vi "AIT 664 - ReadWrite All Data.vi"(0 "RT Data in":T2 {"End System Handle" format="%x"; "Label Transfer Config"."Block Data Refs"."Data Reference" format="%.0x"; "Status Config"."Hardware Out Dur Reference" format="%.0x"; "Status Config"."Hardware In Dur Reference" format="%.0x"; "Status Config"."Hardware Out Count Reference" format="%.0x"; "Status Config"."Hardware In Count Reference" format="%.0x"; "Status Config"."Error Data Reference" format="%.0x"; "Hardware Output Tx Channels"."Message Settings"."Transmit Channel Data Reference" format="%.0x"; "Hardware Output Tx Channels"."Message Settings"."Queue Transmit Channel" format="%.0x"; "Hardware Output Tx Channels"."Message Settings"."Driver Data"."Num Bits" min=1 max=32; "Hardware Output Tx Channels"."Message Settings"."Block Data Refs"."Data Reference" format="%.0x"; "Hardware Output Tx Channels"."Rx Com Udp Port"."Handle" format="%08x"; "Hardware Output Tx Channels"."Tx Com Udp Port"."Handle" format="%08x"; "Hardware Input Rx Channels"."Message Settings"."Transmit Channel Data Reference" format="%.0x"; "Hardware Input Rx Channels"."Message Settings"."Queue Transmit Channel" format="%.0x"; "Hardware Input Rx Channels"."Message Settings"."Driver Data"."Num Bits" min=1 max=32; "Hardware Input Rx Channels"."Message Settings"."Block Data Refs"."Data Reference" format="%.0x"; "Hardware Input Rx Channels"."Rx Com Udp Port"."Handle" format="%08x"; "Hardware Input Rx Channels"."Tx Com Udp Port"."Handle" format="%08x"}, 2 "Mode":T1, 5 "Channel Index":i32, 11 "error in (no error)":errorcluster, 12 "Iteration":i32) -> (4 "RT Data out":T2 {"End System Handle" format="%x"; "Label Transfer Config"."Block Data Refs"."Data Reference" format="%.0x"; "Status Config"."Hardware Out Dur Reference" format="%.0x"; "Status Config"."Hardware In Dur Reference" format="%.0x"; "Status Config"."Hardware Out Count Reference" format="%.0x"; "Status Config"."Hardware In Count Reference" format="%.0x"; "Status Config"."Error Data Reference" format="%.0x"; "Hardware Output Tx Channels"."Message Settings"."Transmit Channel Data Reference" format="%.0x"; "Hardware Output Tx Channels"."Message Settings"."Queue Transmit Channel" format="%.0x"; "Hardware Output Tx Channels"."Message Settings"."Driver Data"."Num Bits" min=1 max=32; "Hardware Output Tx Channels"."Message Settings"."Block Data Refs"."Data Reference" format="%.0x"; "Hardware Output Tx Channels"."Rx Com Udp Port"."Handle" format="%08x"; "Hardware Output Tx Channels"."Tx Com Udp Port"."Handle" format="%08x"; "Hardware Input Rx Channels"."Message Settings"."Transmit Channel Data Reference" format="%.0x"; "Hardware Input Rx Channels"."Message Settings"."Queue Transmit Channel" format="%.0x"; "Hardware Input Rx Channels"."Message Settings"."Driver Data"."Num Bits" min=1 max=32; "Hardware Input Rx Channels"."Message Settings"."Block Data Refs"."Data Reference" format="%.0x"; "Hardware Input Rx Channels"."Rx Com Udp Port"."Handle" format="%08x"; "Hardware Input Rx Channels"."Tx Com Udp Port"."Handle" format="%08x"}, 15 "error out":errorcluster)   [LabVIEW 2013, in "AIT 664 Custom Device.lvlib"]
doc: "Given the mode provide either the hardware input or output channels to read/write from hardware or read/write to veristand."
uses:
  AIT 664 Custom Device.lvlib
  RT Controls/AIT 664  - RT Data.ctl
  RT Controls/AIT 664 - RT Hardware Channel.ctl
  RT Controls/AIT 664 - RT Message Settings.ctl
  <vilib>/NI Veristand/Custom Device API/Block Data Reference.ctl
  <vilib>/NI Veristand/Custom Device API/Data Reference.ctl
  RT Controls/AIT 664 - Driver Data.ctl
  Controls and Global/Start Bit.ctl
  Controls and Global/Number of Bits.ctl
  <vilib>/NI Veristand/Custom Device API/Custom Device Item Ref.ctl
  <userlib>/ARINC 664/AIT 664 Controls/General/Message Port.ctl
  <userlib>/ARINC 664/AIT 664 Controls/General/Direction.ctl
  <userlib>/ARINC 664/AIT 664 Controls/General/Message Port Type.ctl
  System Explorer/Controls/664 - Sampling Type.ctl
  RT Controls/Status Channels Config.ctl
  RT Controls/FIFO.ctl
  RT Controls/Label Transfer Config.ctl
  RT Controls/ReadWrite Selector.ctl
  <vilib>/NI Veristand/Custom Device API/Custom Device API.lvlib
  <userlib>/ARINC 664/AIT 664 API.lvlib
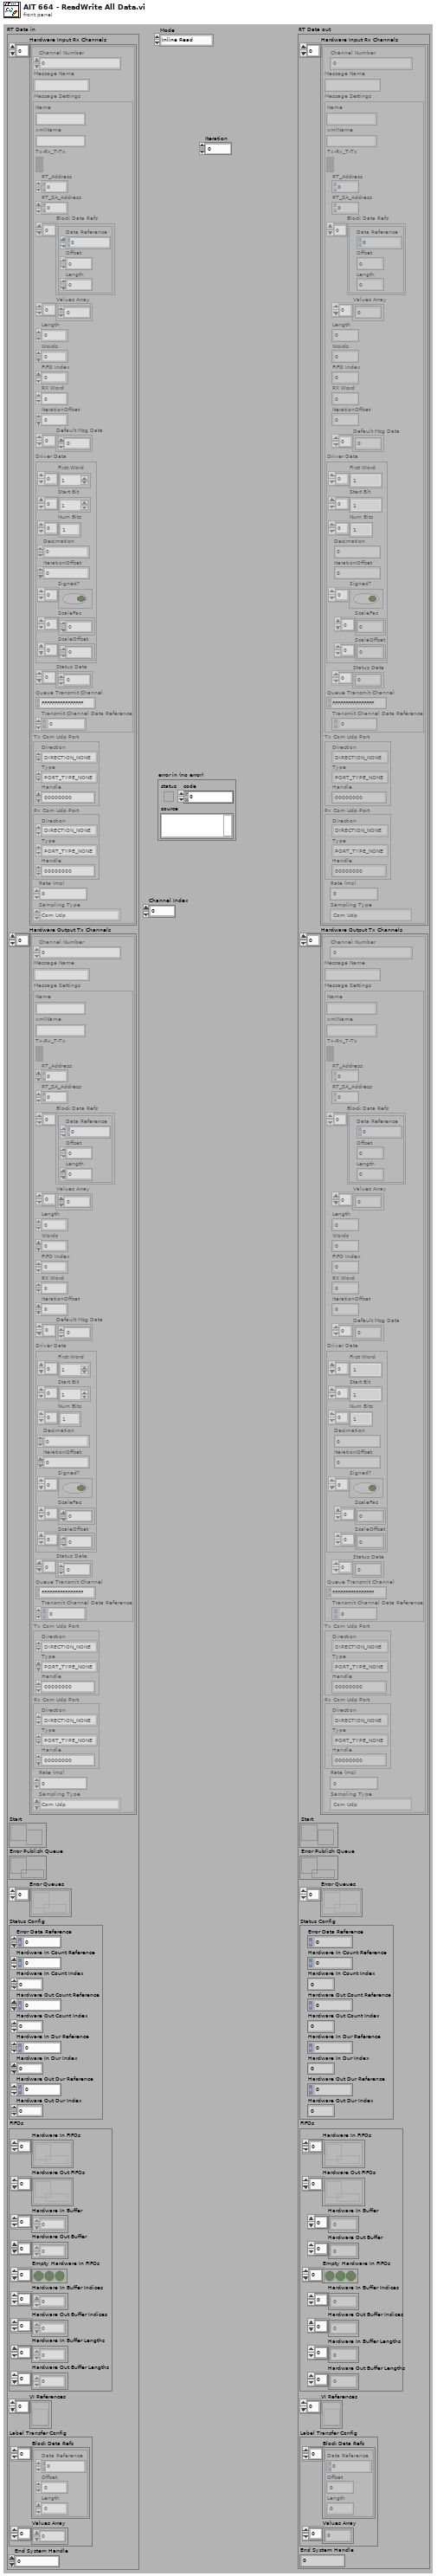
[diagram p1: front panel]
types:
  T1 = typedef "AIT 664 Custom Device.lvlib/ReadWrite Selector.ctl" = enum16{"Inline Read", "Inline Write", "Async HWIn", "Async HWOut"}
  T2 = typedef "AIT 664 Custom Device.lvlib/AIT 664  - RT Data.ctl" = cluster{"Hardware Input Rx Channels":T3[], "Hardware Output Tx Channels":T3[], "Start":refnum<notifier>, "Error Publish Queue":refnum<queue>, "Error Queues":refnum<queue>[], "Status Config":T15, "FIFOs":T16, "VI References":refnum<vi>[], "Label Transfer Config":T17, "End System Handle ":u64}
  T3 = typedef "AIT 664 Custom Device.lvlib/AIT 664 - RT Hardware Channel.ctl" = cluster{"Channel Number":u16, "Message Name":string, "Message Settings":T4, "Tx Com Udp Port":T11, "Rx Com Udp Port":T11, "Rate (ms)":u32, "Sampling Type":T14}
  T4 = typedef "AIT 664 Custom Device.lvlib/AIT 664 - RT Message Settings.ctl" = cluster{"Name":string, "xmlName":string, "Tx-Rx_T-Tx":bool, "RT_Address":u8, "RT_SA_Address":u8, "Block Data Refs":T5[], "Values Array":dbl[], "Length":i32, "Words":i32, "FIFO Index":i32, "RX Word":u32, "IterationOffset":i32, "Default Msg Data":u8[], "Driver Data":T7, "Status Data":u32[], "Queue Transmit Channel":T10, "Transmit Channel Data Reference":T6}
  T5 = typedef "Custom Device API.lvlib/Block Data Reference.ctl" = cluster{"Data Reference":T6, "Offset":i32, "Length":i32}
  T6 = typedef "Custom Device API.lvlib/Data Reference.ctl" = i32
  T7 = typedef "AIT 664 Custom Device.lvlib/AIT 664 - Driver Data.ctl" = cluster{"First Word":T8[], "Start Bit":T8[], "Num Bits":T9[], "Decimation":i32, "IterationOffset":i32, "Signed?":bool[], "ScaleFac":dbl[], "ScaleOffset":dbl[]}
  T8 = typedef "AIT 664 Custom Device.lvlib/Start Bit.ctl" = i32
  T9 = typedef "AIT 664 Custom Device.lvlib/Number of Bits.ctl" = i32
  T10 = typedef "Custom Device API.lvlib/Custom Device Item Ref.ctl" = u64
  T11 = typedef "AIT 664 API.lvlib/Message Port.ctl" = cluster{"Direction":T12, "Type":T13, "Handle":u64}
  T12 = typedef "AIT 664 API.lvlib/Direction.ctl" = enum16{"DIRECTION_NONE", "DIRECTION_TX", "DIRECTION_RX"}
  T13 = typedef "AIT 664 API.lvlib/Message Port Type.ctl" = enum16{"PORT_TYPE_NONE", "COM_UDP", "SAP_UDP", "SAP_IP", "SAP_MAC", "COTS_MAC", "COTS_MAC_RAW"}
  T14 = typedef "AIT 664 Custom Device.lvlib/664 - Sampling Type.ctl" = enum16{"Com Udp", "Com Udp Queuing", "Sap Udp", "Sap Ip", "Sap Mac", "Unknown"}
  T15 = typedef "AIT 664 Custom Device.lvlib/Status Channels Config.ctl" = cluster{"Error Data Reference":T6, "Hardware In Count Reference":T6, "Hardware In Count Index":i32, "Hardware Out Count Reference":T6, "Hardware Out Count Index":i32, "Hardware In Dur Reference":T6, "Hardware In Dur Index":i32, "Hardware Out Dur Reference":T6, "Hardware Out Dur Index":i32}
  T16 = typedef "AIT 664 Custom Device.lvlib/FIFO.ctl" = cluster{"Hardware In FIFOs":refnum<k33>[], "Hardware Out FIFOs":refnum<k33>[], "Hardware In Buffer":dbl[], "Hardware Out Buffer":dbl[], "Empty Hardware In FIFOs":bool[], "Hardware In Buffer Indices":i32[], "Hardware Out Buffer Indices":i32[], "Hardware In Buffer Lengths":i32[], "Hardware Out Buffer Lengths":i32[]}
  T17 = typedef "AIT 664 Custom Device.lvlib/Label Transfer Config.ctl" = cluster{"Block Data Refs":T5[], "Values Array":dbl[]}
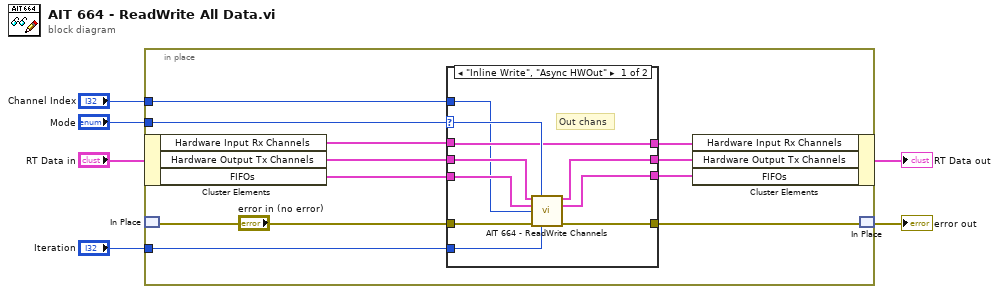
[diagram p0: block diagram]
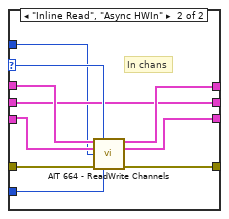
[diagram p2: hidden frame]
diagram:
  n1 = in-place {
    in-place-border: "Mode" -> [w12]
    in-place-border: "Channel Index" -> [w9]
    in-place-border: "Iteration" -> [w8]
    n2 = in-place-cluster #1("RT Data in") -> ("Hardware Input Rx Channels"=w18:T3[], "Hardware Output Tx Channels"=w11:T3[], "FIFOs"=w14:T16)
    n3 = in-place-match #2("error in (no error)") -> (w16:errorcluster)
    n4 = case shown="\"Inline Write\", \"Async HWOut\"" w12 {
      selector: w12 -> [w27 w34]
      tunnel: w18 -> [w23 w38]
      tunnel: [w23 w37] -> w17
      tunnel: w16 -> [w28 w36]
      tunnel: [w26 w35] -> w15
      tunnel: w14 -> [w21 w32]
      tunnel: [w22 w31] -> w13
      tunnel: w11 -> [w25 w33]
      tunnel: [w24 w33] -> w10
      tunnel: w9 -> [w19 w29]
      tunnel: w8 -> [w20 w30]
      frame "Inline Write", "Async HWOut" {
        # "Out chans"
        n5 = call "AIT 664 - ReadWrite Channels.vi"("Channels In"=w25, "Mode"=w27, "FIFOs In"=w21, "Channel Index"=w19, "error in (no error)"=w28, "Iteration"=w20) -> ("Channels Out"=w24:T3[], "FIFOs Out"=w22:T16, "error out"=w26:errorcluster)  [unwired: 7 in]
      }
      frame "Inline Read", "Async HWIn" {
        # "In chans"
        n6 = call "AIT 664 - ReadWrite Channels.vi"("Channels In"=w38, "Mode"=w34, "FIFOs In"=w32, "Channel Index"=w29, "error in (no error)"=w36, "Iteration"=w30) -> ("Channels Out"=w37:T3[], "FIFOs Out"=w31:T16, "error out"=w35:errorcluster)  [unwired: 7 in]
      }
    }
    n7 = in-place-cluster #1("Hardware Input Rx Channels"=w17, "Hardware Output Tx Channels"=w10, "FIFOs"=w13) -> (→"RT Data out":T2)
    n8 = in-place-match #2(w15) -> (→"error out":errorcluster)
  }
